vi "SetAdGain_thread.vi"(1 "gain":u8=6, 2 "board_sel":u32=1) -> ()   [LabVIEW 2015]
uses:
  ESLSCDLL.dll
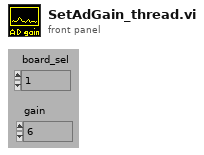
[diagram p1: front panel]
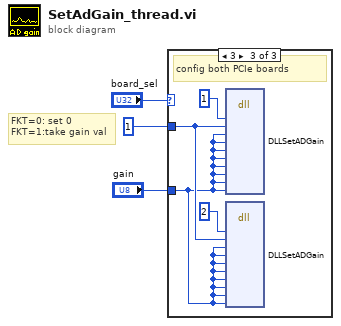
[diagram p0: block diagram]
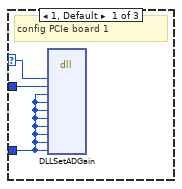
[diagram p2: hidden frame]
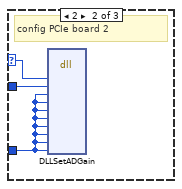
[diagram p3: hidden frame]
diagram:
  # "FKT=0: set 0\nFKT=1:take gain val"
  n1 = case shown="3" "board_sel" {
    selector: "board_sel" -> [w6 w9 _]
    tunnel: u8 1 -> [w5 w8 w11]
    tunnel: "gain" -> [w4 w7 w10]
    frame 1, Default {
      # "config PCIe board 1"
      n2 = dll-call lib="C:/ENTW/PCIE/lv64/board.vis/ESLSCDLL.dll" fn="DLLSetADGain" ("lwlscdll.dll:DLLSetADAmpRed")("drv"=w6, "fkt"=w5, "g1"=w4, "g2"=w4, "g3"=w4, "g4"=w4, "g5"=w4, "g6"=w4, "g7"=w4, "g8"=w4) -> ()  [unwired: 14 in, 2 out]
    }
    frame 2 {
      # "config PCIe board 2"
      n3 = dll-call lib="C:/ENTW/PCIE/lv64/board.vis/ESLSCDLL.dll" fn="DLLSetADGain" ("lwlscdll.dll:DLLSetADAmpRed")("drv"=w9, "fkt"=w8, "g1"=w7, "g2"=w7, "g3"=w7, "g4"=w7, "g5"=w7, "g6"=w7, "g7"=w7, "g8"=w7) -> ()  [unwired: 14 in, 2 out]
    }
    frame 3 {
      # "config both PCIe boards"
      n4 = dll-call lib="C:/ENTW/PCIE/lv64/board.vis/ESLSCDLL.dll" fn="DLLSetADGain" ("lwlscdll.dll:DLLSetADAmpRed")("drv"=u32 1, "fkt"=w11, "g1"=w10, "g2"=w10, "g3"=w10, "g4"=w10, "g5"=w10, "g6"=w10, "g7"=w10, "g8"=w10) -> ()  [unwired: 14 in, 2 out]
      n5 = dll-call lib="C:/ENTW/PCIE/lv64/board.vis/ESLSCDLL.dll" fn="DLLSetADGain" ("lwlscdll.dll:DLLSetADAmpRed")("drv"=u32 2, "fkt"=w11, "g1"=w10, "g2"=w10, "g3"=w10, "g4"=w10, "g5"=w10, "g6"=w10, "g7"=w10, "g8"=w10) -> ()  [unwired: 14 in, 2 out]
    }
  }
